vi "Configure FFT Measurement (Channel Power).vi"(8 "error in (no error)":errorcluster, 10 "Measurement Source (0: Function 1)":i32(ring) items=["Function 1", "Function 2", "Function 3", "Function 4", "Math 1", "Math 2", "Math 3", "Math 4", "FFT"], 11 "VISA resource name":refnum<visa-resource-name>) -> (0 "error out":errorcluster, 3 "VISA resource name out":refnum<visa-resource-name>)   [LabVIEW 2017, in "Agilent 2000 3000 X-Series.lvlib"]
doc: "Configures FFT analysis channel power measurement.\n\n<b>Note:</b>\n - This VI is only applicable for 3000T, 3000G, 4000, 6000 X-Series.\n - You need to call <b>Configure Math Function Source</b> set the signal source, and call <b>Configure Math Function Characteristics</b>set the function operation mode to FFT and turn on the display of the function."
uses:
  Agilent 2000 3000 X-Series.lvlib
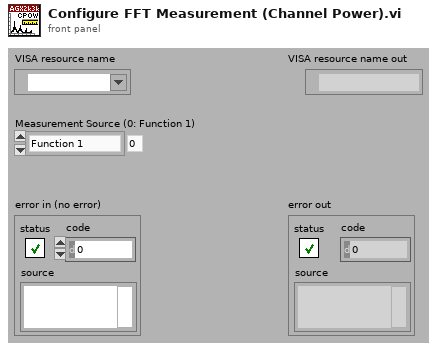
[diagram p1: front panel]
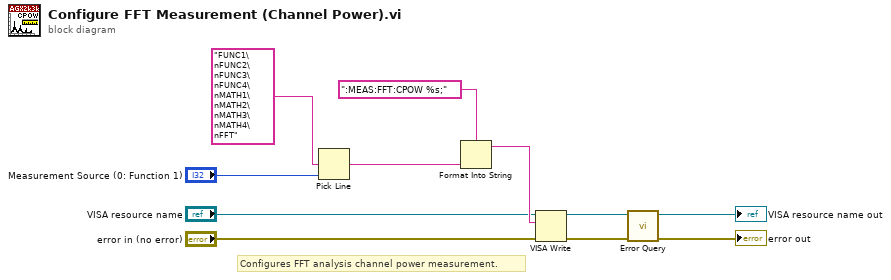
[diagram p0: block diagram]
diagram:
  # "Configures FFT analysis channel power measurement."
  n1 = Pick Line(multi-line string="FUNC1\nFUNC2\nFUNC3\nFUNC4\nMATH1\nMATH2\nMATH3\nMATH4\nFFT", line index="Measurement Source (0: Function 1)") -> (output string=w5:string)  [unwired: 1 in]
  n2 = Format Into String(format string=":MEAS:FFT:CPOW %s;", w5) -> (resulting string=w10:string)  [unwired: 2 in, 1 out]
  n3 = VISA Write(VISA resource name="VISA resource name", write buffer=w10, error in (no error)="error in (no error)") -> (VISA resource name out=w4:refnum<visa-resource-name>, error out=w3:errorcluster)  [unwired: 1 out]
  n4 = call "Error Query.vi"("error in (no error)"=w3, "VISA resource name"=w4) -> ("error out"=→"error out":errorcluster, "VISA resource name out"=→"VISA resource name out":refnum<visa-resource-name>)  [unwired: 6 in, 2 out]
